vi "SRDG535.set Status.vi"(0 "i ref in":refnum<vi>, 5 "error in":errorcluster) -> (14 "i ref out":refnum<vi>, 19 "error out":errorcluster)   [LabVIEW 2014, in "SRDG535.lvlib"]
doc: "This VI sets the status: In case of a device failure it is set to failure (3), otherwise to on (2). The status is indicated and published a DIM-service."
uses:
  SRDG535.lvlib
  CS_PHELIX/PH_Basics/PH_StatusHandler/PH_StatusHandler.Status.ctl
  CS_PHELIX/PH_Basics/PH_StatusHandler/PH_StatusHandler.lvlib
  CSlibraries-extern/DimLVEvent/LVDimInterface/LVDimInterface.lvlib
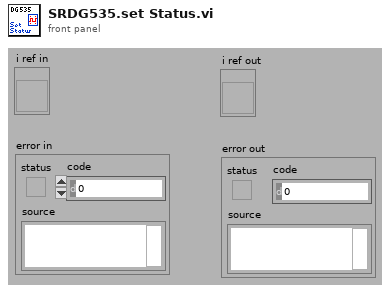
[diagram p1: front panel]
types:
  T1 = typedef "PH_StatusHandler.lvlib/PH_StatusHandler.Status.ctl" = i16
  T2 = typedef "SRDG535.lvlib/SRDG535.i attribute.ctl" = cluster{"GPIB address":string, "Device error":errorcluster, "GUI Refs":cluster{"Delete":refnum<vi>, "Device Error":refnum<vi>, "Information":refnum<vi>, "Output":refnum<vi>, "Delay":refnum<vi>, "Trigger":refnum<vi>}, "Output Settings":T3, "Service ID Rate":i32, "Service IDs Channelinfo":i32[], "Delay Settings":T5, "Trigger Settings":T6}
  T3 = typedef "SRDG535.lvlib/SRDG535.Output.ctl" = cluster{"CH T0":T4, "CH A":T4, "CH B":T4, "CH AB":T4, "CH C":T4, "CH D":T4, "CH CD":T4}
  T4 = typedef "SRDG535.lvlib/SRDG535.Channel Output.ctl" = cluster{"Inversion":bool, "Amplitude (V)":dbl, "Offset (V)":dbl, "Mode":i32, "Load":bool}
  T5 = typedef "SRDG535.lvlib/SRDG535.Delay.ctl" = cluster{"CH A":cluster{"rel to":u32, "Delay (s)":dbl}, "CH B":cluster{"rel to":u32, "Delay (s)":dbl}, "CH C":cluster{"rel to":u32, "Delay (s)":dbl}, "CH D":cluster{"rel to":u32, "Delay (s)":dbl}}
  T6 = typedef "SRDG535.lvlib/SRDG535.Trigger.ctl" = cluster{"trigger":u32, "Impedance":bool, "Slope":bool, "burst count":i32, "external level (V)":sgl, "Internal/Burst Rate (Hz)":dbl, "Burst Period":i32}
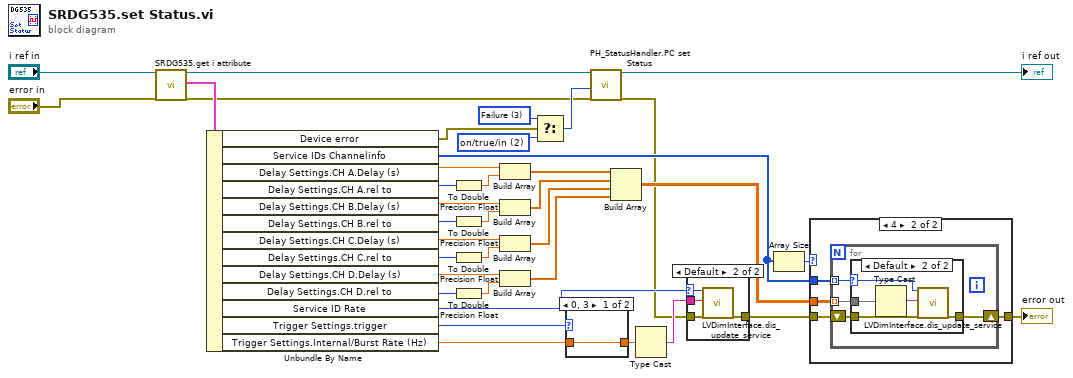
[diagram p0: block diagram]
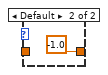
[diagram p5: hidden frame]
diagram:
  w36 = T1 2 items=["no info", "off/false/out", "on/true/in", "Failure", "Alarm", "Status 1", "Status 2", "Status 3"] ("f")
  w35 = T1 3 items=["no info", "off/false/out", "on/true/in", "Failure", "Alarm", "Status 1", "Status 2", "Status 3"] ("Status")
  n1 = call "SRDG535.get i attribute.vi"("i ref in"="i ref in", "error in (no error)"="error in") -> ("i ref out"=w2:refnum<vi>, "i attribute"=w34:T2, "error out"=w8:errorcluster)  [unwired: 15 in]
  n2 = Unbundle By Name(w34) -> ("Device error"=w3:errorcluster, "Service IDs Channelinfo"=w6:i32[], "Delay Settings.CH A.Delay (s)"=w18:dbl, "Delay Settings.CH A.rel to"=w23:u32, "Delay Settings.CH B.Delay (s)"=w17:dbl, "Delay Settings.CH B.rel to"=w22:u32, "Delay Settings.CH C.Delay (s)"=w16:dbl, "Delay Settings.CH C.rel to"=w21:u32, "Delay Settings.CH D.Delay (s)"=w20:dbl, "Delay Settings.CH D.rel to"=w24:u32, "Service ID Rate"=w27:i32, "Trigger Settings.trigger"=w28:u32, "Trigger Settings.Internal/Burst Rate (Hz)"=w29:dbl)
  n3 = To Double Precision Float(number=w23) -> (double precision float=w15:dbl)
  n4 = To Double Precision Float(number=w22) -> (double precision float=w14:dbl)
  n5 = To Double Precision Float(number=w21) -> (double precision float=w13:dbl)
  n6 = To Double Precision Float(number=w24) -> (double precision float=w19:dbl)
  n7 = Build Array(w18, w15) -> (w12:dbl[])
  n8 = Build Array(w17, w14) -> (w11:dbl[])
  n9 = Build Array(w16, w13) -> (w10:dbl[])
  n10 = Build Array(w20, w19) -> (w9:dbl[])
  n11 = Select(t=w35, s=w3, f=w36) -> (s? t:f=w37:T1)
  n12 = case shown="0, 3" w28 {
    tunnel: w29 -> [w38 _]
    tunnel: [w38 -1.0 ("d64")] -> w30
    frame 0, 3 {
    }
    frame Default {
    }
  }
  n13 = call "PH_StatusHandler.PC set Status.vi"("i ref in"=w2, "Status"=w37, "error in (no error)"=w8) -> ("i ref out"=→"i ref out":refnum<vi>, "error out"=w4:errorcluster)  [unwired: 15 in]
  n14 = Build Array(w12, w11, w10, w9) -> (w7:dbl[][])
  n15 = Type Cast(x=w30) -> (*(type *) &x=w31:string)  [unwired: 1 in]
  n16 = case shown="Default" w27 {
    selector: w27 -> [_ w41]
    tunnel: w4 -> [w40 w44]
    tunnel: [w40 w43] -> w25
    tunnel: w31 -> [_ w42]
    frame -1 {
    }
    frame Default {
      n17 = call "LVDimInterface.dis_update_service.vi"("my_serviceID"=w41, "data"=w42, "error in (no error)"=w44) -> ("error out"=w43:errorcluster)  [unwired: 14 in, 2 out]
    }
  }
  n18 = Array Size(array=w6) -> (size(s)=w5:i32)
  n19 = case shown="4" w5 {
    tunnel: [w45 w49] -> w26
    tunnel: w25 -> [w45 w48]
    tunnel: w7 -> [_ w47]
    tunnel: w6 -> [_ w46]
    frame Default {
    }
    frame 4 {
      n20 = for {
        shift-right: [w53] -> w49
        shift-left: w48 -> [w52]
        tunnel: w46 -> [w51] mode=indexing
        tunnel: w47 -> [w50] mode=indexing
        n21 = case shown="Default" w51 {
          selector: w51 -> [_ w55]
          tunnel: [w54 w58] -> w53
          tunnel: w52 -> [w54 w57]
          tunnel: w50 -> [_ w56]
          frame -1 {
          }
          frame Default {
            n22 = Type Cast(x=w56) -> (*(type *) &x=w59:string)  [unwired: 1 in]
            n23 = call "LVDimInterface.dis_update_service.vi"("my_serviceID"=w55, "data"=w59, "error in (no error)"=w57) -> ("error out"=w58:errorcluster)  [unwired: 14 in, 2 out]
          }
        }
      }
    }
  }
  "error out" <- w26
